vi "Get Signal Units by ID.vi"(8 "error in":errorcluster, 11 "PackageID":i32) -> (0 "error out":errorcluster, 3 "Signal Units":string[](array[string]))   [LabVIEW 2021, in "XNET-CAN-Signal-Logger.lvlib"]
uses:
  XNET-CAN-Signal-Logger.lvlib
  Global Variables.vi
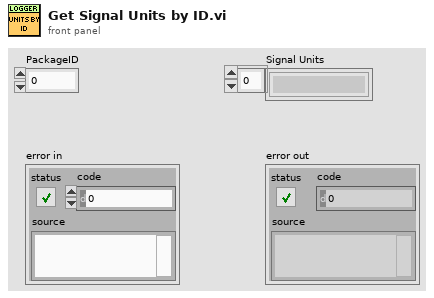
[diagram p1: front panel]
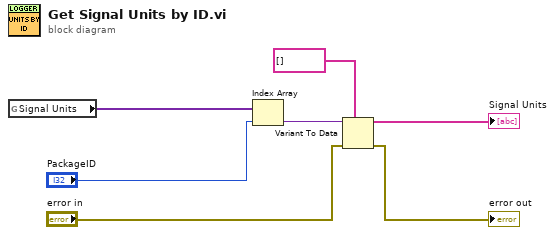
[diagram p0: block diagram]
diagram:
  n1 = global read "Global Variables.vi" "Signal Units"() -> (w7:variant[])
  n2 = Index Array(array=w7, index="PackageID") -> (element=w5:variant)
  n3 = Variant To Data(error in="error in", type=string[] [], Variant=w5) -> (data=→"Signal Units":string[], error out=→"error out":errorcluster)
